vi "Swing Up Energy Control.vi"(2 "u_max (m/s^2)":dbl=6.0 min=0.0 max=10.0 step=0.5, 3 "mu (m/s^2/J)":dbl=50.0 min=0.0 max=150.0 step=5.0, 4 "Er (mJ)":dbl=10.0 min=0.0 max=50.0 step=5.0, 5 "alpha_full (rad)":dbl) -> (0 "E (mJ)":dbl, 1 "u (A)":dbl)   [LabVIEW 2016]
uses:
  <vilib>/Simulation/Implementation/Shared/SIMSCR Execution Mode.ctl
  <vilib>/Simulation/Scripting/Companion Diagram/SimConfigNode/SimParams.ctl
  <vilib>/Simulation/Scripting/Companion Diagram/SimConfigNode/_simSolvers.ctl
  <vilib>/Simulation/Param Hierarchy/Typedefs/SIMPH Param Control Actions.ctl
  <vilib>/Simulation/Implementation/Shared/NILVSim_ParamChanged.vi
  <vilib>/Simulation/Implementation/Shared/NILVSIM_BeginStep.vi
  <vilib>/Simulation/ContinuousLinear/Implementation/NILVSim Transfer Function Direct.llb/SIM Transfer Function Direct (SISO).vi
  <vilib>/Simulation/Nonlinear/Implementation/NILVSim Saturation.llb/SIM Saturation (scalar).vi
  <vilib>/Simulation/Implementation/Shared/NILVSim_Manager.vi
  <vilib>/Utility/error.llb/Clear Errors.vi
  <vilib>/Simulation/Implementation/Shared/NILVSim_FinalizeModel.vi
  <vilib>/Simulation/Implementation/Shared/SIM Unbundle Sim Info.vi
  <vilib>/Simulation/Implementation/Shared/SIMSH Read Queue.vi
  <vilib>/Simulation/Implementation/Shared/NILVSim_Initialize.vi
  <vilib>/Simulation/Utility/Implementation/NILVSim Get Time and IsAcceptedStep.vi
  <vilib>/Simulation/Implementation/Shared/NILVSim_GetModelError.vi
  <vilib>/Simulation/Implementation/Shared/SIM SimErrorHandler.vi
  <vilib>/Simulation/Implementation/Shared/SIM Bundle Sim Info.vi
  <vilib>/Simulation/Scripting/Companion Diagram/SimConfigNode/SimDog.xnode
  <vilib>/Simulation/Implementation/XNodeFramework/SimXNode/SimX.xnode
  <vilib>/Simulation/Implementation/Shared/NI_SIM_Implementation.lvlib
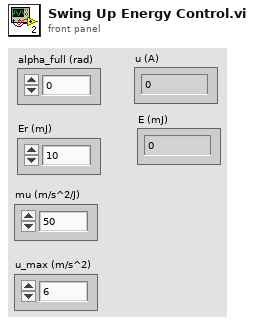
[diagram p1: front panel]
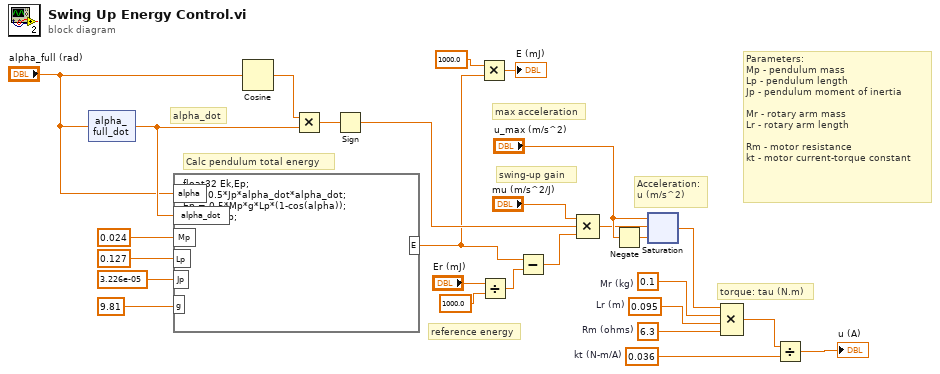
[diagram p0: block diagram]
diagram:
  w24 = 0.036  # kt (N-m/A)
  w22 = 6.3  # Rm (ohms)
  w11 = 0.095  # Lr (m)
  w10 = 0.1  # Mr (kg)
  # "reference energy"
  # "max acceleration"
  # "swing-up gain"
  # "Parameters:\nMp - pendulum mass\nLp - pendulum length\nJp - pendulum moment of inertia\n\nMr - rotary arm mass\nLr - rotary arm length\n\nRm - motor resistance\nkt - motor current-torque constant"
  # "alpha_dot"
  # "Calc pendulum total energy"
  # "Acceleration:\nu (m/s^2)"
  # "torque: tau (N.m)"
  n1 = xnode "alpha_full_dot"("input u(t)"="alpha_full (rad)") -> ("output y(t)"=w14:dbl)  [unwired: 4 in, 1 out]
  n2 = formula code="float32 Ek,Ep;\nEk = 0.5*Jp*alpha_dot*alpha_dot;\nEp = 0.5*Mp*g*Lp*(1-cos(alpha));\nE = Ek+Ep;"("Mp"=0.024 ("input variable"), "Jp"=3.226e-05 ("input variable 3"), "g"=9.81 ("input variable 4"), "Lp"=0.127 ("input variable 2"), "alpha"="alpha_full (rad)", "alpha_dot"=w14) -> ("E"=w3:dbl)
  n3 = Cosine(x="alpha_full (rad)") -> (cos(x)=w13:dbl)
  n4 = Multiply(x=w13, y=w14) -> (x*y=w4:dbl)
  n5 = Sign(1:w4) -> (0:w5:dbl)
  n6 = Multiply ("Multiply 2")(x=1000.0, y=w3) -> (x*y=→"E (mJ)":dbl)
  n7 = Divide ("Divide 2")(x="Er (mJ)", y=1000.0) -> (x/y=w21:dbl)
  n8 = Subtract(x=w3, y=w21) -> (x-y=w6:dbl)
  n9 = Compound Arithmetic op=MULTIPLY("mu (m/s^2/J)", w5, w6) -> (w7:dbl)
  n10 = Negate(x="u_max (m/s^2)") -> (-x=w8:dbl)
  n11 = xnode ("Saturation")("upper limit"="u_max (m/s^2)", "input"=w7, "lower limit"=w8) -> ("output"=w9:dbl)  [unwired: 2 in]
  n12 = Compound Arithmetic op=MULTIPLY ("Compound Arithmetic 2")(w9, w10, w11, w22) -> (w23:dbl)
  n13 = Divide(x=w23, y=w24) -> (x/y=→"u (A)":dbl)
